vi "serial communication to linear card EXAMPLE.vi"() -> ()   [LabVIEW 2012]
doc: "SciScan 1.2 160622"
uses:
  <vilib>/Instr/_visa.llb/VISA Configure Serial Port (Instr).vi
panel:
  out "read buffer":string
  in  "write buffer":string
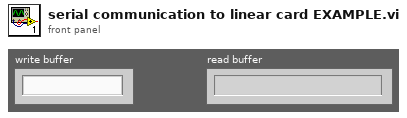
[diagram p1: front panel]
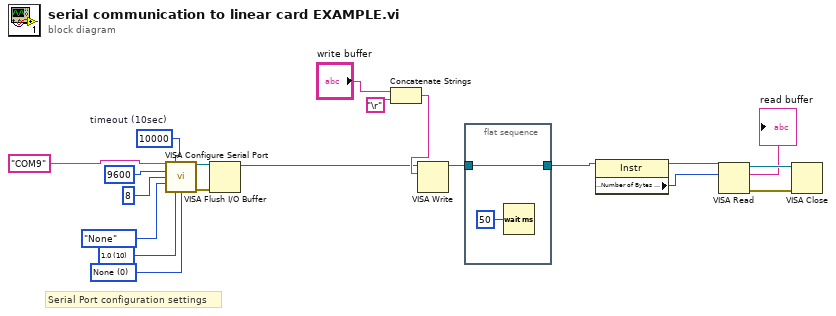
[diagram p0: block diagram]
diagram:
  w18 = u16 0 items=["None", "XON/XOFF", "RTS/CTS", "XON/XOFF & RTS/CTS", "DTR/DSR", "XON/XOFF & DTR/DSR"] ("flow control (0:none)")
  w17 = u16 10 items=["1.0"=10, "1.5"=15, "2.0"=20] ("stop bits (10: 1 bit)")
  w13 = u32 10000  # timeout (10sec)
  # "Serial Port configuration settings"
  n1 = call-poly "VISA Configure Serial Port"("VISA resource name"="COM9" ("write buffer"), "timeout (10sec)"=w13, "baud rate (9600)"=u32 9600, "data bits (8)"=u16 8, "parity (0:none)"=enum16{"None", "Odd", "Even", "Mark", "Space"}."None", "stop bits (10: 1 bit)"=w17, "flow control (0:none)"=w18) -> ("VISA resource name out"=w19:refnum<visa-resource-name>, "error out"=w20:errorcluster)  [unwired: 7 in]
  n2 = VISA Flush I/O Buffer(VISA resource name=w19, error in (no error)=w20) -> (VISA resource name out=w1:refnum<visa-resource-name>)  [unwired: 1 in, 1 out]
  n3 = Concatenate Strings("write buffer", "\r") -> (w2:string)
  n4 = VISA Write(VISA resource name=w1, write buffer=w2) -> (VISA resource name out=w10:refnum<visa-resource-name>)  [unwired: 1 in, 2 out]
  n5 = flat-sequence {
    tunnel: [w21] -> w11
    tunnel: w10 -> [w21]
    frame #0 {
      n6 = Wait (ms)(milliseconds to wait=u32 50) -> ()  [unwired: 1 out]
    }
  }
  n7 = property class="Instr"(reference=w11) -> (reference out=w9:refnum<visa-resource-name>, "Serial Settings:Number of Bytes at Serial Port"=w12:u32)  [unwired: 1 in, 1 out]
  n8 = VISA Read(VISA resource name=w9, byte count=w12) -> (VISA resource name out=w7:refnum<visa-resource-name>, read buffer=→"read buffer":string, error out=w8:errorcluster)  [unwired: 1 in, 1 out]
  n9 = VISA Close(VISA resource name=w7, error in (no error)=w8) -> ()  [unwired: 1 out]
